vi "SelectNetwork.vi"(11 "base path":path) -> (0 "SimPars":T1, 3 "Cerebellum out":refnum<class "Cerebellum.lvclass">)   [LabVIEW 2016]
uses:
  Cerebellum/Cerebellum.lvclass
panel:
  in  "run":bool
  in  "Existing Grids in Results/ 2":i32(listbox)
  out "preview 2":string
  out "preview":string
  in  "Existing Grids in Results/":i32(listbox)
  in  "AERs for LEFT":i32(listbox)
  in  "AERs for RIGHT":i32(listbox)
  # "Select the Networks"
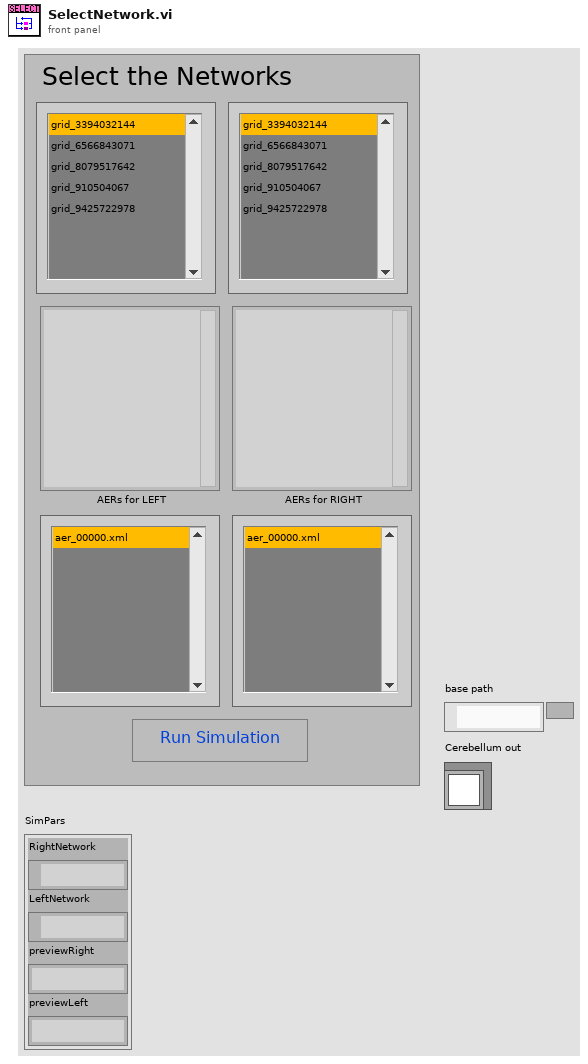
[diagram p1: front panel]
types:
  T1 = cluster{"RightNetwork":path, "LeftNetwork":path, "previewRight":string, "previewLeft":string}
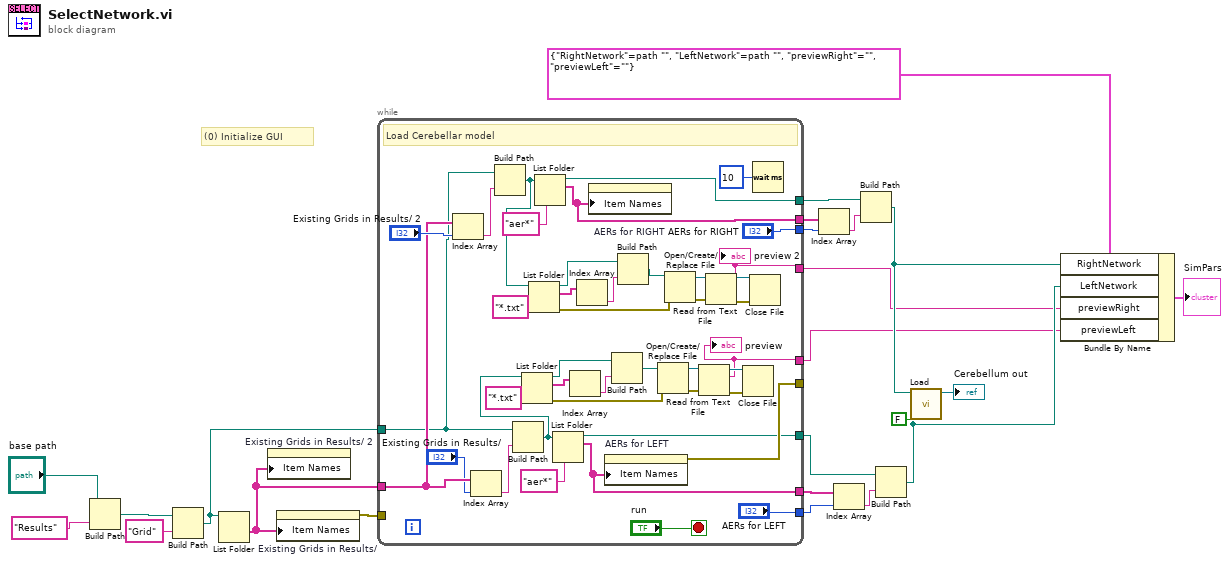
[diagram p0: block diagram]
diagram:
  # "(0) Initialize GUI"
  n1 = Build Path(base path="base path", name or relative path="Results") -> (appended path=w21:path)
  n2 = Build Path(base path=w21, name or relative path="Grid") -> (appended path=w19:path)
  n3 = List Folder(path=w19) -> (folder names=w17:string[])  [unwired: 3 in, 3 out]
  n4 = property on="Existing Grids in Results/ 2" class="LstBox (strict)"("Item Names"=w17) -> ()  [unwired: 2 in, 2 out]
  n5 = property on="Existing Grids in Results/" class="LstBox (strict)"("Item Names"=w17) -> (error out=w20:errorcluster)  [unwired: 2 in, 1 out]
  n6 = while {
    tunnel: w20 -> [_]
    tunnel: w17 -> [w58]
    tunnel: w19 -> [w56]
    tunnel: [w62] -> _
    tunnel: [w61] -> w11
    tunnel: [w31] -> w12
    tunnel: [w30] -> w16
    tunnel: [w29] -> w14
    tunnel: ["AERs for LEFT"] -> w10
    tunnel: ["AERs for RIGHT"] -> w9
    tunnel: [w25] -> w2
    tunnel: [w24] -> w3
    stop <- "run" stop-if-true
    # "Load Cerebellar model"
    n7 = Index Array(array=w58, index="Existing Grids in Results/ 2") -> (element=w57:string)
    n8 = Index Array(array=w58, index="Existing Grids in Results/") -> (element=w64:string)
    n9 = Build Path(base path=w56, name or relative path=w57) -> (appended path=w48:path)
    n10 = Build Path(base path=w56, name or relative path=w64) -> (appended path=w37:path)
    n11 = List Folder(path=w37, pattern="*.txt") -> (path out=w34:path, filenames=w42:string[], error out=w40:errorcluster)  [unwired: 2 in, 1 out]
    n12 = List Folder(path=w48, pattern="*.txt") -> (path out=w45:path, filenames=w46:string[], error out=w49:errorcluster)  [unwired: 2 in, 1 out]
    n13 = List Folder(path=w48, pattern="aer*") -> (path out=w29:path, filenames=w30:string[])  [unwired: 2 in, 2 out]
    n14 = List Folder(path=w37, pattern="aer*") -> (path out=w61:path, filenames=w31:string[])  [unwired: 2 in, 2 out]
    n15 = Index Array(array=w42) -> (element=w35:string)  [unwired: 1 in]
    n16 = Index Array(array=w46) -> (element=w44:string)  [unwired: 1 in]
    n17 = property on="AERs for RIGHT" class="LstBox (strict)"("Item Names"=w30) -> ()  [unwired: 2 in, 2 out]
    n18 = property on="AERs for LEFT" class="LstBox (strict)"("Item Names"=w31) -> (error out=w62:errorcluster)  [unwired: 2 in, 1 out]
    n19 = Build Path(base path=w34, name or relative path=w35) -> (appended path=w36:path)
    n20 = Build Path(base path=w45, name or relative path=w44) -> (appended path=w43:path)
    n21 = Open/Create/Replace File(file path (use dialog)=w36, error in=w40) -> (refnum out=w32:refnum<file>, error out=w38:errorcluster)  [unwired: 4 in, 1 out]
    n22 = Open/Create/Replace File(file path (use dialog)=w43, error in=w49) -> (refnum out=w54:refnum<file>, error out=w55:errorcluster)  [unwired: 4 in, 1 out]
    n23 = Read from Text File(file (use dialog)=w32, error in=w38) -> (refnum out=w33:refnum<file>, text=w25:string, error out=w39:errorcluster)  [unwired: 2 in, 1 out]
    "preview" <- w25
    n24 = Read from Text File(file (use dialog)=w54, error in=w55) -> (refnum out=w52:refnum<file>, text=w24:string, error out=w53:errorcluster)  [unwired: 2 in, 1 out]
    "preview 2" <- w24
    n25 = Close File(refnum=w33, error in=w39) -> ()  [unwired: 2 out]
    n26 = Close File(refnum=w52, error in=w53) -> ()  [unwired: 2 out]
    n27 = Wait (ms)(milliseconds to wait=u32 10) -> ()  [unwired: 1 out]
  }
  n28 = Index Array(array=w16, index=w9) -> (element=w15:string)
  n29 = Index Array(array=w12, index=w10) -> (element=w13:string)
  n30 = Build Path(base path=w14, name or relative path=w15) -> (appended path=w5:path)
  n31 = Build Path(base path=w11, name or relative path=w13) -> (appended path=w4:path)
  n32 = call "Load.vi"("Trained?"=FALSE, "Left Hem Path"=w4, "Right Hem Path"=w5) -> ("Cerebellum out"=→"Cerebellum out":refnum<class "Cerebellum.lvclass">)  [unwired: 8 in]
  n33 = Bundle By Name(cluster=T1 {"RightNetwork"=path "", "LeftNetwork"=path "", "previewRight"="", "previewLeft"=""}, "RightNetwork"=w5, "LeftNetwork"=w4, "previewRight"=w3, "previewLeft"=w2) -> (→"SimPars":T1)
